vi "SPI RX bytes.vi"(11 "I/O Cluster In":T1) -> (1 "Output Byte":bool[](array[boolean]), 3 "I/O Cluster Out":T1)   [LabVIEW 2018, in "jmslib.lvlib"]
uses:
  jmslib.lvlib
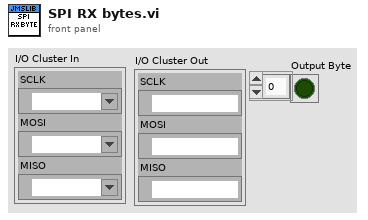
[diagram p1: front panel]
types:
  T1 = cluster{"SCLK":refnum<k21>, "MOSI":refnum<k21>, "MISO":refnum<k21>}
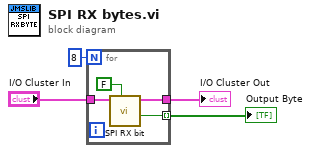
[diagram p0: block diagram]
diagram:
  n1 = for {
    N: 8 ("y") -> [_]
    tunnel: [w8] -> w4 mode=indexing
    tunnel: "I/O Cluster In" -> [w5]
    tunnel: [w6] -> w1
    n2 = call "SPI RX bit.vi"("CPOL"=FALSE ("Falling Edge?"), "I/O Cluster In"=w5) -> ("Signal"=w8:bool, "I/O Cluster Out"=w6:T1)  [unwired: 8 in]
  }
  "Output Byte" <- w4
  "I/O Cluster Out" <- w1
